vi "MOKE_lock-in input sweep_1022D.vi"() -> ()   [LabVIEW 2022 SP3]
uses:
  <vilib>/Analysis/baseanly.llb/Mean (DBL).vi
  <vilib>/Utility/file.llb/Write Delimited Spreadsheet (DBL).vi
  <vilib>/Analysis/NI_AALBase.lvlib
panel:
  in  "Step Size [ms]":i32
  in  "Test Duration [s]":i32
  out "XY Graph 2":cluster{dbl[], dbl[]}(graph)
  out "XY Graph":cluster{dbl[], dbl[]}(graph)
  out "XY Graph 4":cluster{dbl[], dbl[]}(graph)
  out "XY Graph 3":cluster{dbl[], dbl[]}(graph)
  out "phase B":dbl
  in  "Phase B":u16(ring)=9 items=["X", "Y", "R", "Theta", "Frequency", "Noise", "Xh1", "Yh1", "Rh1", "Theta h1", "Xh2", "Yh2", "Rh2", "Theta h2"]
  out "phase A":dbl
  in  "Phase A":u16(ring)=3 items=["X", "Y", "R", "Theta", "Frequency", "Noise", "Xh1", "Yh1", "Rh1", "Theta h1", "Xh2", "Yh2", "Rh2", "Theta h2"]
  out "para1 Measurement":dbl=1.49013e-07
  in  "Clear Plot A":bool
  in  "Parameter A":u16(ring)=2 items=["X", "Y", "R", "Theta", "Frequency", "Noise", "Xh1", "Yh1", "Rh1", "Theta h1", "Xh2", "Yh2", "Rh2", "Theta h2"]
  out "para2 Measurement":dbl=1.49013e-07
  in  "Clear Plot B":bool
  in  "Parameter B":u16(ring)=8 items=["X", "Y", "R", "Theta", "Frequency", "Noise", "Xh1", "Yh1", "Rh1", "Theta h1", "Xh2", "Yh2", "Rh2", "Theta h2"]
  in  "lockin waiting (s)":dbl=0.1 format="%#_13g"
  in  "Save data or not":bool=TRUE
  in  "Series Resistance":string="20kOhm"
  in  "Temperature \n& Field Function":bool
  in  "Field Approach":i32(ring) items=["Linear", "NoOvershoot", "Oscillate"]
  in  "F Rate (Oe/s)":dbl=100.0 format="%#_13g"
  in  "Set F (Oe)":dbl format="%#_13g"
  in  "Mode":i32(ring) items=["Persistent", "Driven"]
  in  "Temperature Approach":i32(ring)=1 items=["FastSettle", "NoOvershoot"]
  in  "T  Rate (K/min)":dbl=10.0
  in  "Set  T  (K)":dbl=2.0
  in  "WaitForField":bool=TRUE
  in  "WaitForTemperature":bool=TRUE
  out "Temperature Status":i32(ring) items=["TemperatureUnknown"=0, "Stable"=1, "Tracking"=2, "Near"=5, "Chasing"=6, "Filling"=7, "Standby"=10, "Disabled"=13, "ImpedanceNotFunction"=14, "TempFailure"=15]
  out "Field Status":i32(ring) items=["MagnetUnknown"=0, "StablePersistent"=1, "WarmingSwitch"=2, "CoolingSwitch"=3, "StableDriven"=4, "Iterating"=5, "Charging"=6, "Discharging"=7, "CurrentError"=8, "MagnetFailure"=15]
  out "Field":dbl
  in  "Delay":dbl=5.0
  out "Temperature":dbl
  in  "Remote":bool=TRUE
  in  "IP Address":string="169.254.170.239"
  out "Measuring":bool
  in  "A Low Pass Filter Slope":u8(ring)=2 items=["6 dB/oct", "12 dB/oct", "18 db/oct", "24 dB/oct"]
  in  "B Low Pass Filter Slope":u8(ring)=2 items=["6 dB/oct", "12 dB/oct", "18 db/oct", "24 dB/oct"]
  in  "B Reference Source":u8(ring)=1 items=["External", "Internal", "Internal Sweep", "Channel-A"]
  in  "B Time Constant":u8(ring)=9 items=["10 us", "30 us", "100 us", "300 us", "1 ms", "3 ms", "10 ms", "30 ms", "100 ms", "300 ms", "1 s", "3 s", "10 s", "30 s", "100 s", "300 s", "1 ks", "3 ks"]
  in  "Enable Sync Filter B (open when f<200Hz)":bool
  in  "B Sensitivity":u16(ring)=17 items=["1 nV/fA", "2 nV/fA", "5 nV/fA", "10 nV/fA", "20 nV/fA", "50 nV/fA", "100 nV/fA", "200 nV/fA", "500 nV/fA", "1 uV/pA", "2 uV/pA", "5 uV/pA", "10 uV/pA", "20 uV/pA", "50 uV/pA", "100 uV/pA", "200 uV/pA", "500 uV/pA", "1 mV/nA", "2 mV/nA", "5 mV/nA", "10 mV/nA", "20 mV/nA", "50 mV/nA", "100 mV/nA", "200 mV/nA", "500 mV/nA", "1 V/uA"]
  in  "A Sensitivity":u16(ring)=23 items=["1 nV/fA", "2 nV/fA", "5 nV/fA", "10 nV/fA", "20 nV/fA", "50 nV/fA", "100 nV/fA", "200 nV/fA", "500 nV/fA", "1 uV/pA", "2 uV/pA", "5 uV/pA", "10 uV/pA", "20 uV/pA", "50 uV/pA", "100 uV/pA", "200 uV/pA", "500 uV/pA", "1 mV/nA", "2 mV/nA", "5 mV/nA", "10 mV/nA", "20 mV/nA", "50 mV/nA", "100 mV/nA", "200 mV/nA", "500 mV/nA", "1 V/uA"]
  in  "Enable Sync Filter A (open when f<200Hz)":bool
  in  "A Time Constant":u8(ring)=9 items=["10 us", "30 us", "100 us", "300 us", "1 ms", "3 ms", "10 ms", "30 ms", "100 ms", "300 ms", "1 s", "3 s", "10 s", "30 s", "100 s", "300 s", "1 ks", "3 ks"]
  in  "B Sample time (s)":dbl=0.001 min=0.001 max=100.0 step=0.001
  in  "A Sample time (s)":dbl=0.001 min=0.001 max=100.0 step=0.001
  in  "stabilization(S)":dbl=1.0 format="%#_13g"
  in  "B frequency":dbl=50063.4 format="%#_13g"
  in  "B Input Connection (0: Single-Ended)":u16(ring) items=["Single-Ended Voltage", "Differential Voltage", "1 MOhm Current Gain", "100 MOhm Current Gain"]
  in  "B harmonic 1":u8=2
  in  "B harmonic 2":u8=3
  in  "B reference Manual Phase  2":dbl=-59.75
  in  "auto phase B":bool=TRUE
  in  "A frequency":dbl=267.77 format="%#_13g"
  in  "A Input Connection (0: Single-Ended)":u16(ring) items=["Single-Ended Voltage", "Differential Voltage", "1 MOhm Current Gain", "100 MOhm Current Gain"]
  in  "A harmonic 1":u8=2
  in  "A harmonic 2":u8=3
  in  "A reference Manual Phase":dbl=-59.75
  in  "auto phase A":bool=TRUE
  in  "A Reference Source":u8(ring) items=["External", "Internal", "Internal Sweep"]
  in  "path (folder + filename)":string="G:\\My Drive\\Opticool\\Measurement\\NLH\\f dependence\\TaI18_a48_b78_17.7Hz"
  in  "LOCKIN address":refnum<visa-resource-name>="COM3"
  # "Lock-in Setting"
  # "Channel B"
  # "Channel A"
  # "Mesurement"
  # "Sine Sweep Setting (Channel A)"
  # "Temprature and Field Setting"
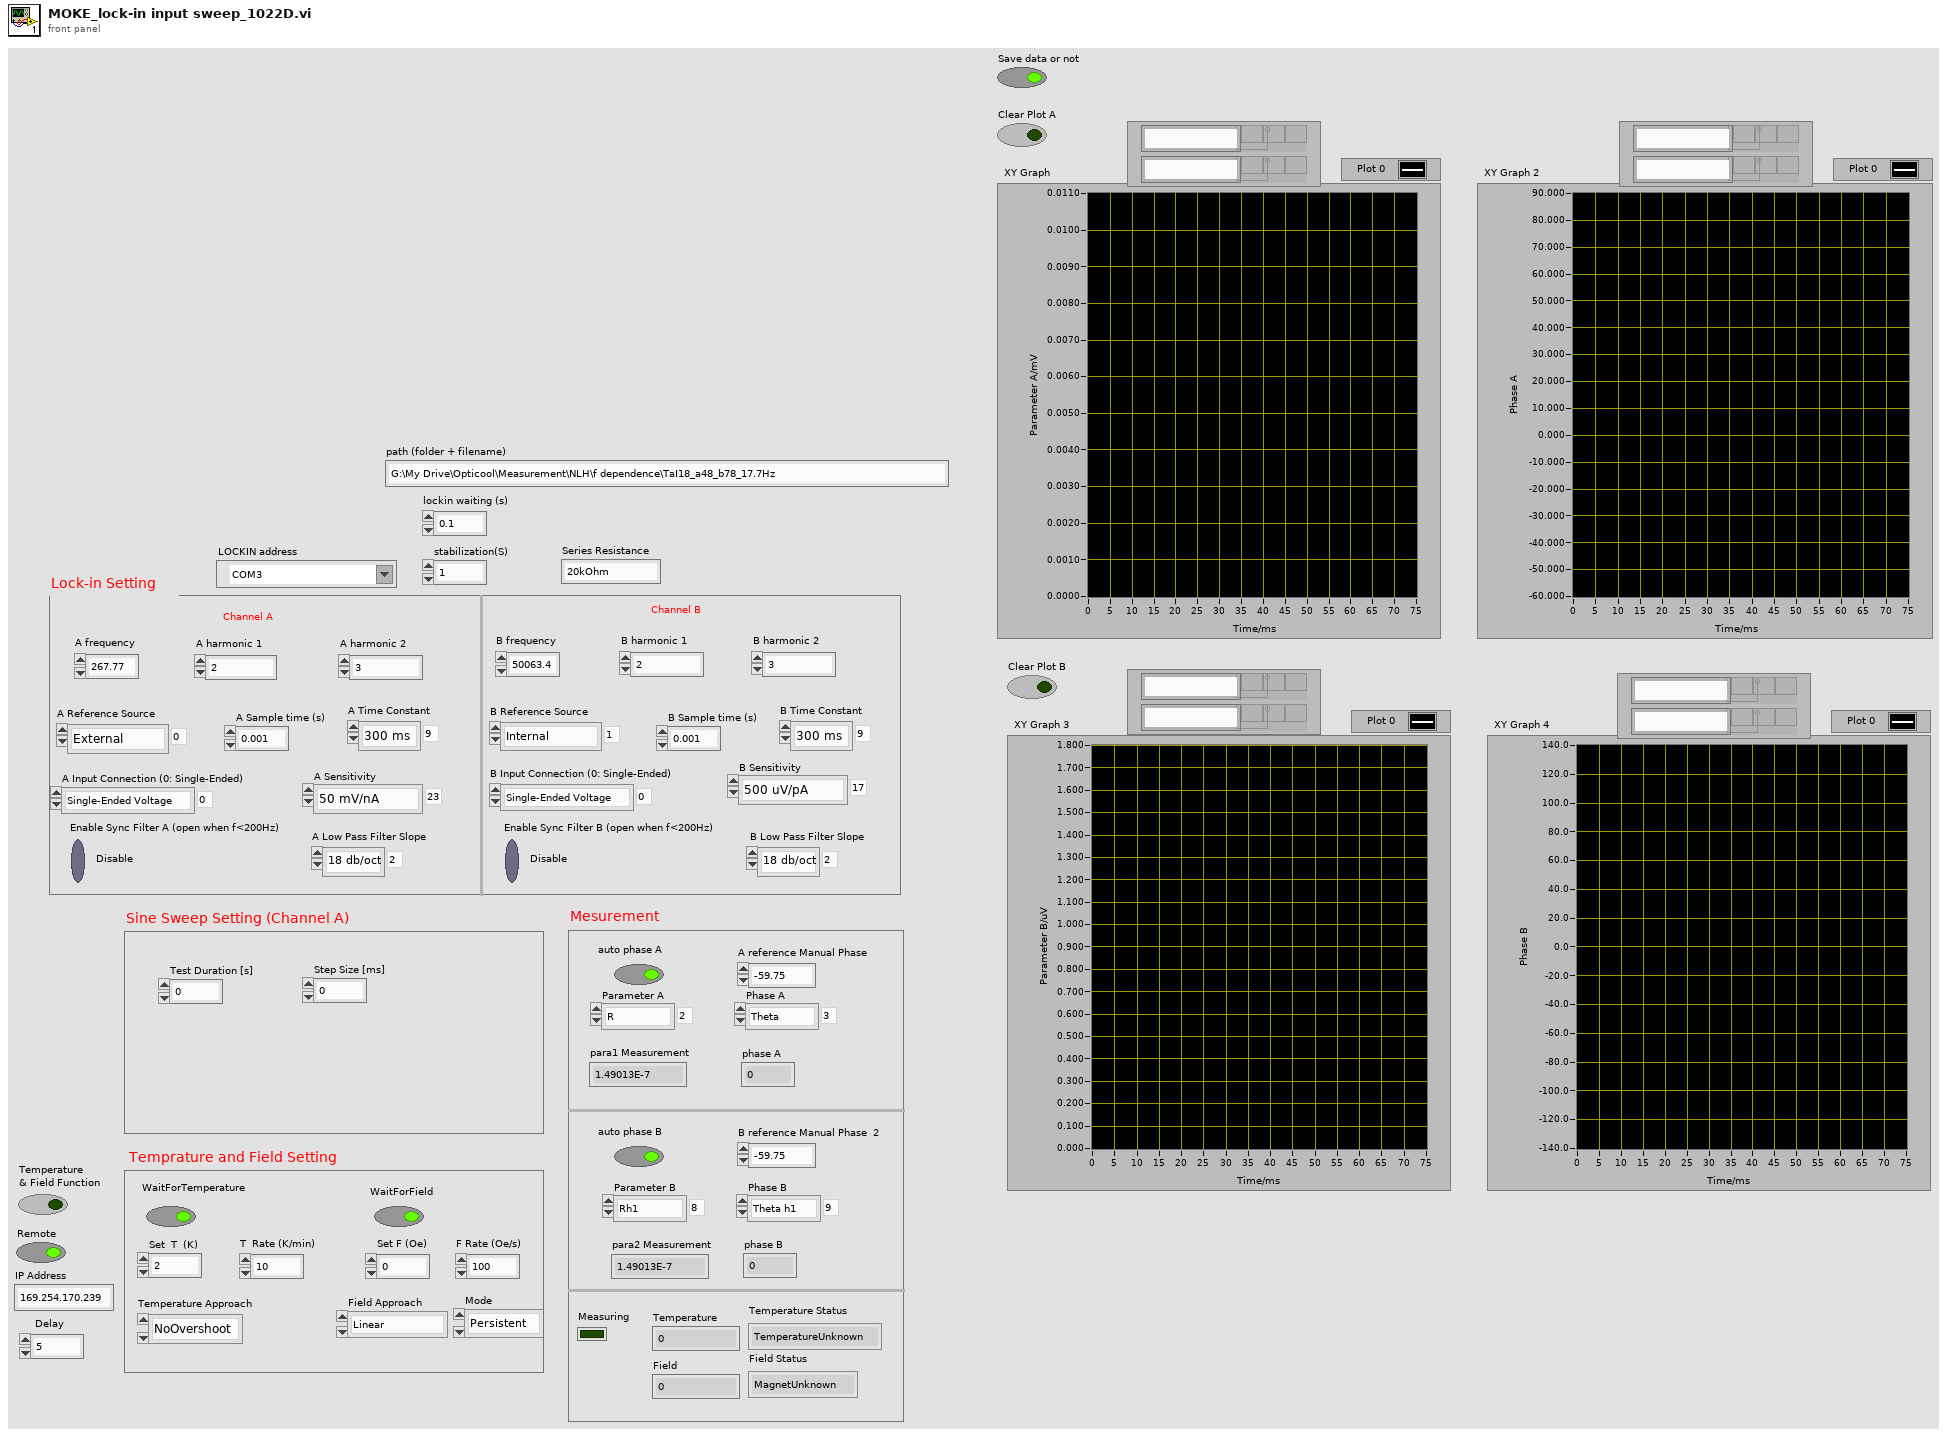
[diagram p1: front panel]
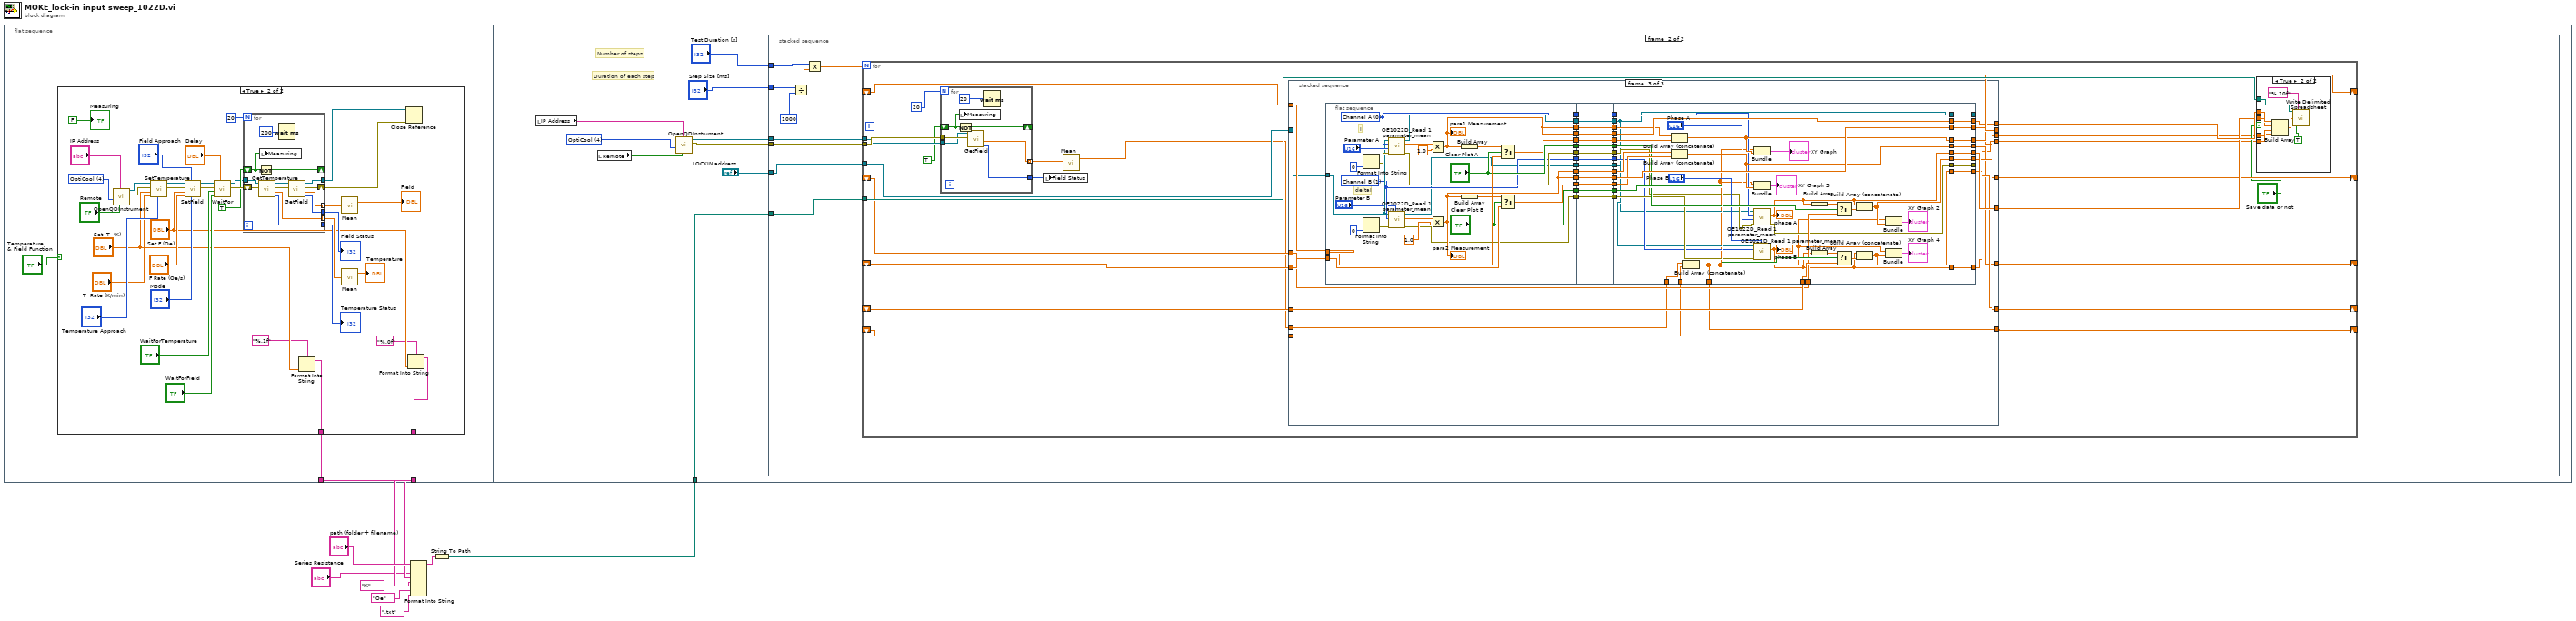
[diagram p0: block diagram]
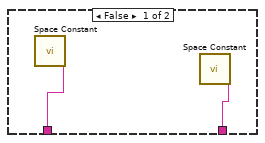
[diagram p2: hidden frame]
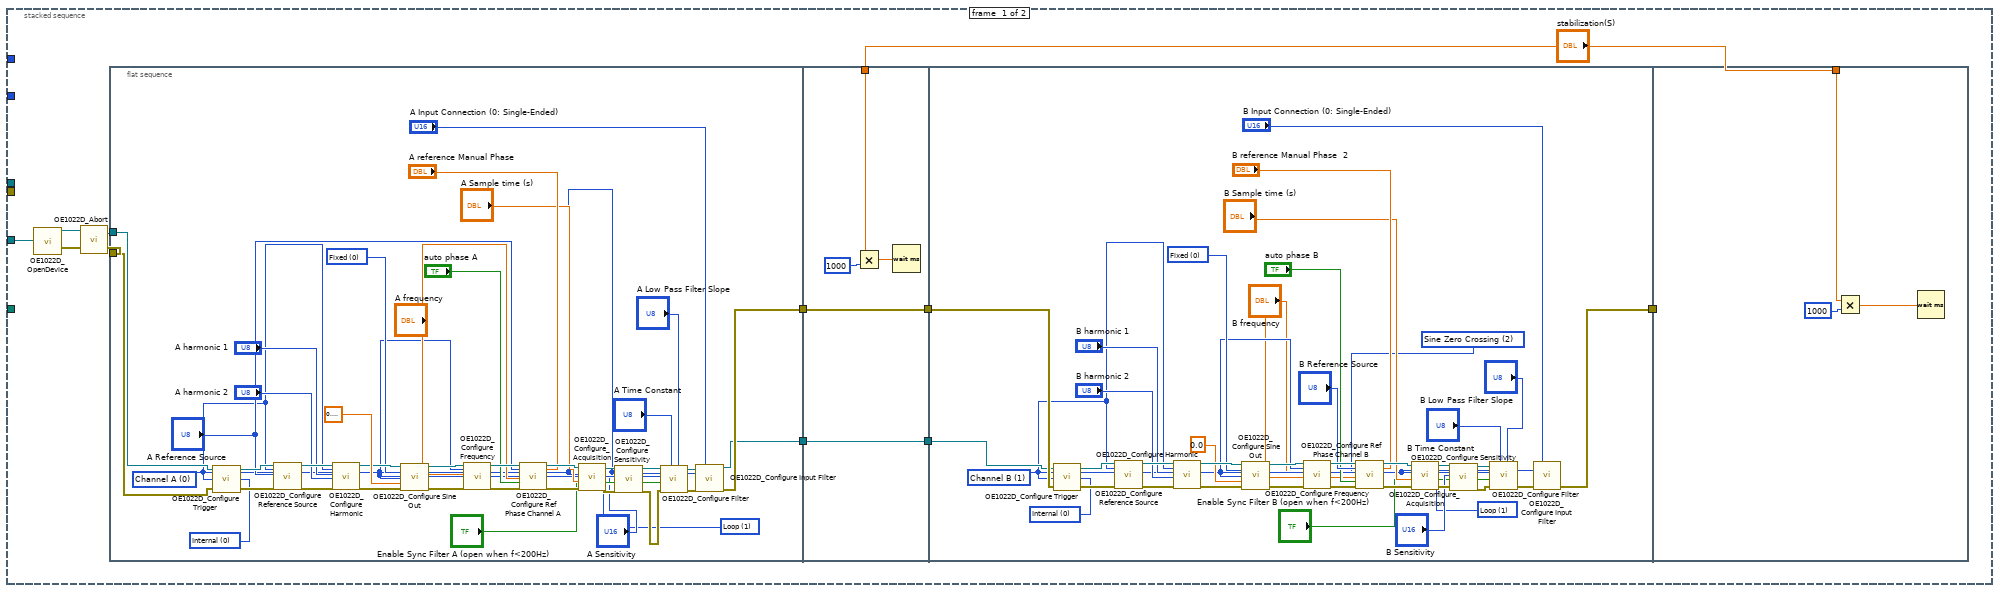
[diagram p3: hidden frame]
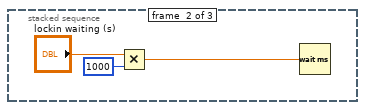
[diagram p6: hidden frame]
diagram:
  n1 = flat-sequence {
    tunnel: [w12] -> w2
    tunnel: [w11] -> w6
    tunnel: w9 -> [w71]
    frame #0 {
      n2 = case shown="True" "Temperature \n& Field Function" {
        tunnel: [w14 w16] -> w12
        tunnel: [w13 w15] -> w11
        frame False {
          n3 = call <vilib>:"Space Constant.vi"() -> ("String"=w14:string)
          n4 = call <vilib>:"Space Constant.vi"() -> ("String"=w13:string)
        }
        frame True {
          w41 = 4 items=["PPMS", "VersaLab", "DynaCool", "SVSM", "OptiCool"] ("InstrumentType")
          n5 = call "OpenQDInstrument.vi"("Remote"="Remote", "IP Address"="IP Address", "InstrumentType"=w41) -> ("error out"=w28:errorcluster, "Instrument Ref"=w29:refnum<k24>)  [unwired: 5 in]
          n6 = call "SetTemperature.vi"("Approach"="Temperature Approach", "Rate"="T  Rate (K/min)", "Temperature"="Set  T  (K)", "error in (no error)"=w28, "Instrument Ref In"=w29) -> ("error out"=w47:errorcluster, "Instrument Ref Out"=w46:refnum<k24>)  [unwired: 2 in, 1 out]
          n7 = call "SetField.vi"("Mode"="Mode", "Approach"="Field Approach", "Rate"="F Rate (Oe/s)", "Field"="Set F (Oe)", "error in (no error)"=w47, "Instrument Ref In"=w46) -> ("error out"=w24:errorcluster, "Instrument Ref Out"=w25:refnum<k24>)  [unwired: 1 in, 1 out]
          n8 = call "WaitFor.vi"("Delay"="Delay", "Wait For Field"="WaitForField", "Wait For Temperature"="WaitForTemperature", "error in (no error)"=w24, "Instrument Ref In"=w25) -> ("error out"=w40:errorcluster, "Instrument Ref Out"=w36:refnum<k24>)  [unwired: 5 in]
          n9 = for {
            N: 20 -> [_]
            shift-right: [w63] -> _
            shift-left: TRUE -> [w61]
            shift-right: [w58] -> w26
            shift-left: w40 -> [w60]
            tunnel: w36 -> [w57]
            tunnel: [w55] -> w27
            tunnel: [w52] -> w35
            tunnel: [w51] -> w34
            tunnel: [w53] -> w32 mode=indexing
            tunnel: [w54] -> w33 mode=indexing
            n10 = Not(x=w61) -> (.not. x?=w63:bool)
            n11 = call "GetTemperature.vi"("error in (no error)"=w60, "Instrument Ref In"=w57) -> ("Temperature\nStatus"=w51:i32, "Temperature"=w54:dbl, "error out"=w59:errorcluster, "Instrument Ref Out"=w56:refnum<k24>)  [unwired: 3 in, 1 out]
            n12 = local write "Measuring"(w61) -> ()
            n13 = Wait (ms)(milliseconds to wait=u32 200) -> ()  [unwired: 1 out]
            n14 = call "GetField.vi"("error in (no error)"=w59, "Instrument Ref In"=w56) -> ("Field\nStatus"=w52:i32, "Field"=w53:dbl, "error out"=w58:errorcluster, "Instrument Ref Out"=w55:refnum<k24>)  [unwired: 3 in, 1 out]
          }
          "Field Status" <- w35
          "Temperature Status" <- w34
          n15 = Format Into String(format string="%.1f", "Set  T  (K)") -> (resulting string=w16:string)  [unwired: 2 in, 1 out]
          n16 = call-poly <vilib>:"Mean.vi"("X"=w32) -> ("mean"=→"Field":dbl)  [unwired: 1 out]
          n17 = call-poly <vilib>:"Mean.vi"("X"=w33) -> ("mean"=→"Temperature":dbl)  [unwired: 1 out]
          n18 = Close Reference(reference=w27, error in (no error)=w26) -> ()  [unwired: 1 out]
          n19 = Format Into String(format string="%.0f", "Set F (Oe)") -> (resulting string=w15:string)  [unwired: 2 in, 1 out]
          "Measuring" <- FALSE
        }
      }
    }
    frame #1 {
      w67 = 4 items=["PPMS", "VersaLab", "DynaCool", "SVSM", "OptiCool"] ("InstrumentType")
      # "Duration of each step"
      # "Number of steps"
      n20 = local read "IP Address"() -> (w66:string)
      n21 = local read "Remote"() -> (w68:bool)
      n22 = call "OpenQDInstrument.vi"("Remote"=w68, "IP Address"=w66, "InstrumentType"=w67) -> ("error out"=w64:errorcluster, "Instrument Ref"=w65:refnum<k24>)  [unwired: 5 in]
      n23 = stacked-sequence {
        tunnel: "LOCKIN address" -> [w75 w176]
        tunnel: w71 -> [_ w177]
        tunnel: "Test Duration [s]" -> [_ w175]
        tunnel: "Step Size [ms]" -> [_ w174]
        tunnel: w65 -> [_ w170]
        tunnel: w64 -> [_ w169]
        frame #0 {
          n24 = call <instrlib>:"OE1022D_OpenDevice.vi"("VISA resource name"=w75) -> ("VISA资源名称输出"=w74:refnum<visa-resource-name>, "错误输出"=w76:errorcluster)  [unwired: 17 in]
          n25 = call <instrlib>:"OE1022D_Abort.vi"("error in (no error)"=w76, "VISA resource name"=w74) -> ("error out"=w81:errorcluster, "VISA resource name out"=w82:refnum<visa-resource-name>)
          n26 = flat-sequence {
            tunnel: w82 -> [w122]
            tunnel: [w110] -> w80
            tunnel: w81 -> [w121]
            tunnel: [w98] -> w78
            tunnel: w80 -> [w127]
            tunnel: [w127] -> w79
            tunnel: w78 -> [w126]
            tunnel: [w126] -> w77
            tunnel: "stabilization(S)" -> [w123]
            tunnel: w79 -> [w148]
            tunnel: [w147] -> w83
            tunnel: w77 -> [w146]
            tunnel: w83 -> [_]
            tunnel: "stabilization(S)" -> [w166]
            frame #0 {
              w84 = u8 1 items=["Single", "Loop"] ("Sample Mode (Single/Loop)")
              w97 = u8 0 items=["Fixed", "Linear", "Log"] ("SineOut Mode")
              w99 = u16 0 items=["Internal", "External"] ("Trigger Source (0: Internal)")
              w88 = u8 0 items=["Channel A", "Channel B"] ("OE1022D A/B")
              n27 = call <instrlib>:"OE1022D_Configure Trigger.vi"("Trigger Source (0: Internal)"=w99, "error in (no error)   2"=w121, "OE1022D A/B"=w88, "VISA resource name   2"=w122) -> ("error out   2"=w115:errorcluster, "VISA resource name out   2"=w116:refnum<visa-resource-name>)
              n28 = call <instrlib>:"OE1022D_Configure Reference Source.vi"("VISA resource name"=w116, "OE1022D A/B"=w88, "Reference Source"="A Reference Source", "error in (no error)"=w115) -> ("VISA resource name out"=w114:refnum<visa-resource-name>, "error out"=w112:errorcluster)  [unwired: 14 in]
              n29 = call <instrlib>:"OE1022D_Configure Harmonic.vi"("VISA resource name"=w114, "OE1022D A/B"=w88, "Harmonic 1"="A harmonic 1", "Harmonic 2"="A harmonic 2", "error in (no error)"=w112) -> ("VISA resource name out"=w113:refnum<visa-resource-name>, "error out"=w111:errorcluster)  [unwired: 13 in]
              n30 = call <instrlib>:"OE1022D_Configure Sine Out.vi"("VISA resource name"=w113, "SineOut Mode"=w97, "OE1022D A/B"=w88, "Sine Output Amplitude (V)"=sgl 0.1, "error in (no error)"=w111) -> ("VISA resource name out"=w119:refnum<visa-resource-name>, "error out"=w118:errorcluster)  [unwired: 9 in]
              n31 = call <instrlib>:"OE1022D_Configure Frequency.vi"("VISA resource name"=w119, "OE1022D A/B"=w88, "Internal Frequency(Hz)"="A frequency", "error in (no error)"=w118) -> ("VISA resource name out"=w109:refnum<visa-resource-name>, "error out"=w106:errorcluster)  [unwired: 14 in]
              n32 = call <instrlib>:"OE1022D_Configure Ref Phase Channel A.vi"("VISA resource name"=w109, "Reference Source"="A Reference Source", "Internal Frequency(Hz)"="A frequency", "Auto Phase (T: Enabled)"="auto phase A", "error in (no error)"=w106, "Manual Phase  (degree)"="A reference Manual Phase") -> ("VISA resource name out"=w108:refnum<visa-resource-name>, "error out"=w107:errorcluster)  [unwired: 12 in]
              n33 = call <instrlib>:"OE1022D_Configure_Acquisition.vi"("VISA resource name"=w108, "OE1022D A/B"=w88, "Sample time (s)"="A Sample time (s)", "error in (no error)"=w107, "Sample Mode (Single/Loop)"=w84) -> ("VISA resource name out"=w91:refnum<visa-resource-name>, "error out"=w90:errorcluster)  [unwired: 3 in]
              n34 = call <instrlib>:"OE1022D_Configure Sensitivity.vi"("VISA resource name"=w91, "OE1022D A/B"=w88, "Sensitivity"="A Sensitivity", "error in (no error)"=w90) -> ("VISA resource name out"=w95:refnum<visa-resource-name>, "error out"=w94:errorcluster)  [unwired: 14 in]
              n35 = call <instrlib>:"OE1022D_Configure Filter.vi"("Low Pass Filter Slope (1: 12dB/oct)"="A Low Pass Filter Slope", "Time Constant (8: 100ms)"="A Time Constant", "error in (no error)"=w94, "Enable Sync Filter (F: Disable)"="Enable Sync Filter A (open when f<200Hz)", "OE1022D A/B"=w88, "VISA resource name"=w95) -> ("error out"=w92:errorcluster, "VISA resource name out"=w93:refnum<visa-resource-name>)  [unwired: 4 in]
              n36 = call <instrlib>:"OE1022D_Configure Input Filter.vi"("VISA resource name"=w93, "Input Source"="A Input Connection (0: Single-Ended)", "OE1022D A/B"=w88, "error in (no error)"=w92) -> ("VISA resource name out"=w98:refnum<visa-resource-name>, "error out"=w110:errorcluster)  [unwired: 10 in]
            }
            frame #1 {
              n37 = Multiply(x=w123, y=1000) -> (x*y=w125:dbl)
              n38 = Wait (ms)(milliseconds to wait=w125) -> ()  [unwired: 1 out]
            }
            frame #2 {
              w128 = u8 1 items=["Single", "Loop"] ("Sample Mode (Single/Loop)")
              w130 = u8 2 items=["TTL Pos", "TTL Neg", "Sine Zero Crossing"] ("External Ref Trigger")
              w143 = u8 0 items=["Fixed", "Linear", "Log"] ("SineOut Mode")
              w149 = u16 0 items=["Internal", "External"] ("Trigger Source (0: Internal)")
              w135 = u8 1 items=["Channel A", "Channel B"] ("OE1022D A/B")
              n39 = call <instrlib>:"OE1022D_Configure Trigger.vi"("Trigger Source (0: Internal)"=w149, "error in (no error)   2"=w148, "OE1022D A/B"=w135, "VISA resource name   2"=w146) -> ("error out   2"=w161:errorcluster, "VISA resource name out   2"=w162:refnum<visa-resource-name>)
              n40 = call <instrlib>:"OE1022D_Configure Reference Source.vi"("VISA resource name"=w162, "OE1022D A/B"=w135, "error in (no error)"=w161) -> ("VISA resource name out"=w160:refnum<visa-resource-name>, "error out"=w158:errorcluster)  [unwired: 15 in]
              n41 = call <instrlib>:"OE1022D_Configure Harmonic.vi"("VISA resource name"=w160, "OE1022D A/B"=w135, "Harmonic 1"="B harmonic 1", "Harmonic 2"="B harmonic 2", "error in (no error)"=w158) -> ("VISA resource name out"=w159:refnum<visa-resource-name>, "error out"=w157:errorcluster)  [unwired: 13 in]
              n42 = call <instrlib>:"OE1022D_Configure Sine Out.vi"("VISA resource name"=w159, "SineOut Mode"=w143, "OE1022D A/B"=w135, "Sine Output Amplitude (V)"=sgl 0.0, "error in (no error)"=w157) -> ("VISA resource name out"=w164:refnum<visa-resource-name>, "error out"=w163:errorcluster)  [unwired: 9 in]
              n43 = call <instrlib>:"OE1022D_Configure Frequency.vi"("VISA resource name"=w164, "OE1022D A/B"=w135, "Internal Frequency(Hz)"="B frequency", "error in (no error)"=w163) -> ("VISA resource name out"=w156:refnum<visa-resource-name>, "error out"=w153:errorcluster)  [unwired: 14 in]
              n44 = call <instrlib>:"OE1022D_Configure Ref Phase Channel B.vi"("VISA resource name"=w156, "Reference Source"="B Reference Source", "External Ref Trigger"=w130, "Internal Frequency(Hz)"="B frequency", "Auto Phase (T: Enabled)"="auto phase B", "error in (no error)"=w153, "Manual Phase  (degree)"="B reference Manual Phase  2") -> ("VISA resource name out"=w155:refnum<visa-resource-name>, "error out"=w154:errorcluster)  [unwired: 11 in]
              n45 = call <instrlib>:"OE1022D_Configure_Acquisition.vi"("VISA resource name"=w155, "OE1022D A/B"=w135, "Sample time (s)"="B Sample time (s)", "error in (no error)"=w154, "Sample Mode (Single/Loop)"=w128) -> ("VISA resource name out"=w136:refnum<visa-resource-name>, "error out"=w137:errorcluster)  [unwired: 3 in]
              n46 = call <instrlib>:"OE1022D_Configure Sensitivity.vi"("VISA resource name"=w136, "OE1022D A/B"=w135, "Sensitivity"="B Sensitivity", "error in (no error)"=w137) -> ("VISA resource name out"=w140:refnum<visa-resource-name>, "error out"=w139:errorcluster)  [unwired: 14 in]
              n47 = call <instrlib>:"OE1022D_Configure Filter.vi"("Low Pass Filter Slope (1: 12dB/oct)"="B Low Pass Filter Slope", "Time Constant (8: 100ms)"="B Time Constant", "error in (no error)"=w139, "Enable Sync Filter (F: Disable)"="Enable Sync Filter B (open when f<200Hz)", "OE1022D A/B"=w135, "VISA resource name"=w140) -> ("error out"=w138:errorcluster)  [unwired: 4 in, 1 out]
              n48 = call <instrlib>:"OE1022D_Configure Input Filter.vi"("Input Source"="B Input Connection (0: Single-Ended)", "OE1022D A/B"=w135, "error in (no error)"=w138) -> ("error out"=w147:errorcluster)  [unwired: 11 in, 1 out]
            }
            frame #3 {
              n49 = Multiply(x=w166, y=1000) -> (x*y=w168:dbl)
              n50 = Wait (ms)(milliseconds to wait=w168) -> ()  [unwired: 1 out]
            }
          }
        }
        frame #1 {
          n51 = Divide(x=w174, y=1000) -> (x/y=w172:dbl)
          n52 = Multiply(x=w175, y=w172) -> (x*y=w171:dbl)
          n53 = for {
            N: w171 -> [_]
            tunnel: w176 -> [w201]
            shift-right: [w193] -> _
            shift-left: _ -> [w200]
            tunnel: w177 -> [w198]
            shift-right: [w196] -> _
            shift-left: _ -> [w195]
            shift-right: [w192] -> _
            shift-left: _ -> [w191]
            shift-right: [w190] -> _
            shift-left: _ -> [w189]
            shift-right: [w186] -> _
            shift-left: _ -> [w185]
            tunnel: w170 -> [w183]
            tunnel: w169 -> [w184]
            n54 = for {
              N: 20 -> [_]
              tunnel: w184 -> [w208]
              tunnel: w183 -> [w207]
              shift-right: [w205] -> _
              shift-left: TRUE -> [w204]
              tunnel: [w203] -> w179 mode=indexing
              tunnel: [w202] -> w180
              n55 = Not(x=w204) -> (.not. x?=w205:bool)
              n56 = local write "Measuring"(w204) -> ()
              n57 = call "GetField.vi"("error in (no error)"=w208, "Instrument Ref In"=w207) -> ("Field\nStatus"=w202:i32, "Field"=w203:dbl)  [unwired: 3 in, 3 out]
              n58 = Wait (ms)(milliseconds to wait=20) -> ()  [unwired: 1 out]
            }
            n59 = local write "Field Status"(w180) -> ()
            n60 = call-poly <vilib>:"Mean.vi"("X"=w179) -> ("mean"=w178:dbl)  [unwired: 1 out]
            n61 = stacked-sequence {
              tunnel: w201 -> [_ _ w271]
              tunnel: w200 -> [_ _ w273]
              tunnel: [_ _ w272] -> w193
              tunnel: [_ _ w270] -> w199
              tunnel: [_ _ w269] -> w197
              tunnel: [_ _ w268] -> w196
              tunnel: w195 -> [_ _ w261]
              tunnel: [_ _ w267] -> w192
              tunnel: w191 -> [_ _ w262]
              tunnel: [_ _ w266] -> w190
              tunnel: w189 -> [_ _ w265]
              tunnel: [_ _ w264] -> w188
              tunnel: [_ _ w263] -> w187
              tunnel: w178 -> [_ _ w222]
              tunnel: [_ _ w221] -> w186
              tunnel: w185 -> [_ _ w220]
              frame #0 {
              }
              frame #1 {
                n62 = Multiply(x="lockin waiting (s)", y=1000) -> (x*y=w219:dbl)
                n63 = Wait (ms)(milliseconds to wait=w219) -> ()  [unwired: 1 out]
              }
              frame #2 {
                n64 = flat-sequence {
                  tunnel: w273 -> [w298]
                  tunnel: w271 -> [w280]
                  tunnel: w265 -> [w292]
                  tunnel: [w296] -> w260
                  tunnel: [w289] -> w258
                  tunnel: [w287] -> w256
                  tunnel: [w289] -> w254
                  tunnel: [w288] -> w252
                  tunnel: [w287] -> w250
                  tunnel: [w286] -> w248
                  tunnel: ["Clear Plot B"] -> w246
                  tunnel: ["Clear Plot A"] -> w244
                  tunnel: [w276] -> w242
                  tunnel: [w278] -> w240
                  tunnel: [w277] -> w238
                  tunnel: [w283] -> w236
                  tunnel: [w282] -> w234
                  tunnel: w260 -> [w314]
                  tunnel: [w314] -> w259
                  tunnel: w258 -> [w313]
                  tunnel: [w313] -> w257
                  tunnel: w256 -> [w312]
                  tunnel: [w312] -> w255
                  tunnel: w254 -> [w311]
                  tunnel: [w311] -> w253
                  tunnel: w252 -> [w310]
                  tunnel: [w310] -> w251
                  tunnel: w250 -> [w309]
                  tunnel: [w309] -> w249
                  tunnel: w248 -> [w308]
                  tunnel: [w308] -> w247
                  tunnel: w246 -> [w307]
                  tunnel: [w307] -> w245
                  tunnel: w244 -> [w306]
                  tunnel: [w306] -> w243
                  tunnel: w242 -> [w305]
                  tunnel: [w305] -> w241
                  tunnel: w240 -> [w304]
                  tunnel: [w304] -> w239
                  tunnel: w238 -> [w303]
                  tunnel: [w303] -> w237
                  tunnel: w236 -> [w302]
                  tunnel: [w302] -> w235
                  tunnel: w234 -> [w301]
                  tunnel: [w301] -> w233
                  tunnel: w259 -> [w325]
                  tunnel: w257 -> [w350]
                  tunnel: w255 -> [w349]
                  tunnel: w253 -> [w347]
                  tunnel: w251 -> [w346]
                  tunnel: w249 -> [w343]
                  tunnel: w247 -> [w342]
                  tunnel: w262 -> [w340]
                  tunnel: w245 -> [w339]
                  tunnel: w261 -> [w337]
                  tunnel: w243 -> [w336]
                  tunnel: w241 -> [w332]
                  tunnel: w239 -> [w331]
                  tunnel: w237 -> [w330]
                  tunnel: w235 -> [w327]
                  tunnel: w233 -> [w326]
                  tunnel: [w325] -> w232
                  tunnel: [w345] -> w231
                  tunnel: [w350] -> w230
                  tunnel: [w323] -> w229
                  tunnel: [w324] -> w228
                  tunnel: [w348] -> w227
                  tunnel: [w344] -> w226
                  tunnel: [w341] -> w225
                  tunnel: [w349] -> w224
                  tunnel: [w329] -> w223
                  tunnel: w222 -> [w320]
                  tunnel: [w319] -> w221
                  tunnel: w220 -> [w318]
                  tunnel: [w351] -> w263
                  tunnel: [w352] -> w264
                  tunnel: [w353] -> w266
                  tunnel: [w354] -> w267
                  tunnel: [w355] -> w268
                  tunnel: [w356] -> _
                  tunnel: [w357] -> w269
                  tunnel: [w358] -> w270
                  tunnel: [w359] -> w272
                  tunnel: [w360] -> _
                  tunnel: w232 -> [w360]
                  tunnel: w231 -> [w359]
                  tunnel: w230 -> [w358]
                  tunnel: w229 -> [w357]
                  tunnel: w228 -> [w356]
                  tunnel: w227 -> [w355]
                  tunnel: w226 -> [w354]
                  tunnel: w225 -> [w353]
                  tunnel: w224 -> [w352]
                  tunnel: w223 -> [w351]
                  frame #0 {
                    w278 = u8 1 items=["Channel A", "Channel B"] ("Channel A/B for Parameter1")
                    w282 = u8 0 items=["Channel A", "Channel B"] ("Channel A/B for Parameter1")
                    # "I"
                    # "deltaI"
                    n65 = Format Into String(0) -> (error out=w297:errorcluster)  [unwired: 3 in, 1 out]
                    n66 = Format Into String(0) -> (error out=w279:errorcluster)  [unwired: 3 in, 1 out]
                    n67 = call <instrlib>:"OE1022D_Read 1 parameter_mean.vi"("错误输入（无错误）"=w297, "Parameter"="Parameter A", "Channel (0: A)"=w282, "VISA resource name"=w280) -> ("error out"=w283:errorcluster, "Measurement"=w290:dbl, "VISA resource name out"=w296:refnum<visa-resource-name>)  [unwired: 5 in]
                    n68 = call <instrlib>:"OE1022D_Read 1 parameter_mean.vi"("Parameter 2"="Parameter B", "错误输入（无错误）"=w279, "Channel (0: A)"=w278, "VISA resource name"=w280) -> ("error out"=w276:errorcluster, "Measurement"=w275:dbl, "VISA resource name out"=w277:refnum<visa-resource-name>)  [unwired: 5 in]
                    n69 = Multiply(x=w290, y=1.0) -> (x*y=w289:dbl)
                    "para1 Measurement" <- w289
                    n70 = Multiply(x=w275, y=1.0) -> (x*y=w287:dbl)
                    "para2 Measurement" <- w287
                    n71 = Build Array(w289) -> (w299:dbl[])
                    n72 = Build Array(w287) -> (w293:dbl[])
                    n73 = Select(t=w299, s="Clear Plot A", f=w298) -> (s? t:f=w288:dbl[])
                    n74 = Select(t=w293, s="Clear Plot B", f=w292) -> (s? t:f=w286:dbl[])
                  }
                  frame #1 {
                  }
                  frame #2 {
                    n75 = Build Array (concatenate)(w347, w346) -> (w345:dbl[])
                    n76 = Build Array (concatenate)(w343, w342) -> (w341:dbl[])
                    n77 = Build Array (concatenate)(w320, w318) -> (w319:dbl[])
                    n78 = Bundle(w319, w345) -> (→"XY Graph":cluster{dbl[], dbl[]})  [unwired: 1 in]
                    n79 = Bundle(w319, w341) -> (→"XY Graph 3":cluster{dbl[], dbl[]})  [unwired: 1 in]
                    n80 = call <instrlib>:"OE1022D_Read 1 parameter_mean.vi"("错误输入（无错误）"=w327, "Parameter"="Phase A", "Channel (0: A)"=w326, "VISA resource name"=w325) -> ("error out"=w324:errorcluster, "Measurement"=w323:dbl)  [unwired: 5 in, 1 out]
                    "phase A" <- w323
                    n81 = call <instrlib>:"OE1022D_Read 1 parameter_mean.vi"("Parameter 2"="Phase B", "错误输入（无错误）"=w332, "Channel (0: A)"=w331, "VISA resource name"=w330) -> ("Measurement"=w329:dbl)  [unwired: 5 in, 2 out]
                    "phase B" <- w329
                    n82 = Build Array(w323) -> (w333:dbl[])
                    n83 = Build Array(w329) -> (w334:dbl[])
                    n84 = Select(t=w333, s=w336, f=w337) -> (s? t:f=w335:dbl[])
                    n85 = Select(t=w334, s=w339, f=w340) -> (s? t:f=w338:dbl[])
                    n86 = Build Array (concatenate)(w323, w335) -> (w348:dbl[])
                    n87 = Build Array (concatenate)(w329, w338) -> (w344:dbl[])
                    n88 = Bundle(w319, w348) -> (→"XY Graph 2":cluster{dbl[], dbl[]})  [unwired: 1 in]
                    n89 = Bundle(w319, w344) -> (→"XY Graph 4":cluster{dbl[], dbl[]})  [unwired: 1 in]
                  }
                  frame #3 {
                  }
                }
              }
            }
            n90 = case shown="True" "Save data or not" {
              tunnel: w199 -> [_ w212]
              tunnel: w198 -> [_ w215]
              tunnel: w197 -> [_ w211]
              tunnel: w188 -> [_ w210]
              tunnel: w187 -> [_ w209]
              frame False {
              }
              frame True {
                n91 = Build Array(w212, w211, w210, w209) -> (w214:dbl[])
                n92 = call-poly <vilib>:"Write Delimited Spreadsheet.vi"("file path (dialog if empty)"=w215, "format (%.3f)"="%.10f", "1D data"=w214, "append to file? (new file:F)"=TRUE) -> ()  [unwired: 10 in, 2 out]
              }
            }
          }
        }
      }
    }
  }
  n93 = Format Into String(initial string="path (folder + filename)", "Series Resistance", w2, "K", w6, "Oe", ".txt") -> (resulting string=w3:string)  [unwired: 2 in, 1 out]
  n94 = String To Path(string=w3) -> (path=w9:path)
